vi "DP-Init Hardware.vi"(0 "State in":T2, 1 "L2":dbl format="%#_13g", 5 "freq":dbl[](array[numeric]), 7 "atten":dbl[](array[numeric]), 9 "flip":bool, 11 "error in (no error)":errorcluster, 12 "ntime":i32, 13 "nfreq":i32) -> (14 "stim":T1, 15 "error out":errorcluster)   [LabVIEW 2020]
uses:
  Typedefs/DP-Runtime State.ctl
  epl-vi-lib/Signal Synthesis VIs/4th Generation/Classes/Gate/Gate.lvclass/Gate.ctl
  e3763c63-dfad-46ca-852a-805909099497.vi
  6524839e-d3bd-4753-b68c-3c0b3b588751.vi
  epl-vi-lib/Signal Synthesis VIs/4th Generation/Common/CommonSig-Apply Ramp (2D).vi
  39a6a7b0-f891-48ff-84db-aba283587dcf.vi
  98cf35c3-bd45-4b05-b00a-4840585587a5.vi
  epl-vi-lib/Signal Synthesis VIs/4th Generation/Common/CommonSig-Apply Ramp (2D).vi/00fa021d-ebe0-42e5-9c35-5538040c7da1.vi
  epl-vi-lib/Signal Synthesis VIs/4th Generation/Classes/Gate/Write Ramp (ms).vi
  epl-vi-lib/Signal Synthesis VIs/4th Generation/Classes/Gate/Write Down (ms).vi
  epl-vi-lib/Signal Synthesis VIs/4th Generation/Classes/Gate/Write Asymmetric.vi
  epl-vi-lib/Signal Synthesis VIs/4th Generation/Classes/Gate/Write Shape.vi
  epl-vi-lib/Signal Synthesis VIs/4th Generation/Classes/Gate/Write Duration (ms).vi
  epl-vi-lib/Signal Synthesis VIs/4th Generation/Classes/Gate/Create.vi
  epl-vi-lib/Signal Synthesis VIs/4th Generation/Classes/Gate/Apply.vi
  epl-vi-lib/PXI DAQ VIs/AODO/AODO-Engine.vi
  epl-vi-lib/PXI DAQ VIs/AIDI/AIDI-Engine.vi
  <vilib>/Analysis/NI_AALBase.lvlib
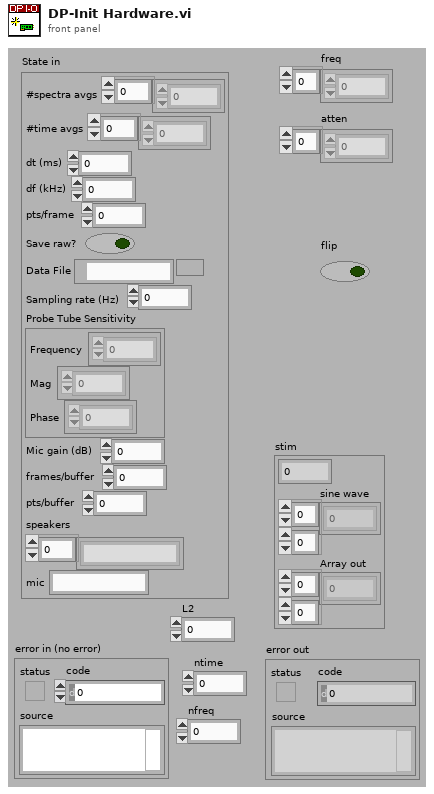
[diagram p1: front panel]
types:
  T1 = cluster{i32, "sine wave":dbl[][], "Array out":dbl[][]}
  T2 = typedef "DP-Runtime State.ctl" = cluster{"#spectra avgs":i32[], "#time avgs":i32[], "dt (ms)":dbl, "df (kHz)":dbl, "pts/frame":i32, "Save raw?":bool, "Data File":path, "Sampling rate (Hz)":dbl, "Probe Tube Sensitivity":cluster{"Frequency":dbl[], "Mag":dbl[], "Phase":dbl[]}, "Mic gain (dB)":dbl, "frames/buffer":i32, "pts/buffer":i32, "speakers":string[], "mic":string}
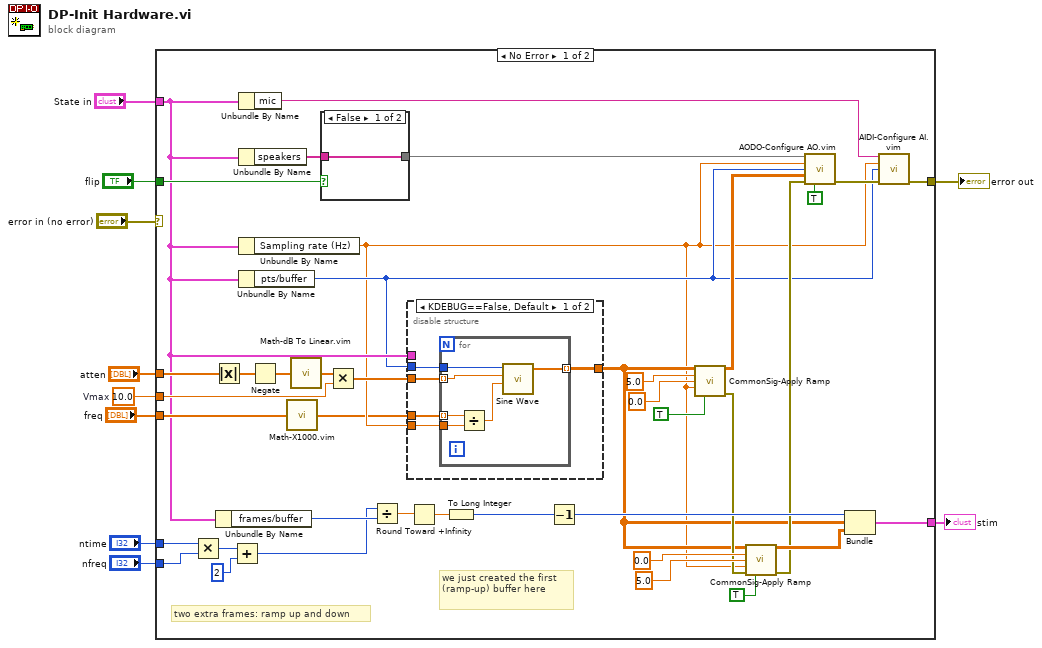
[diagram p0: block diagram]
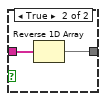
[diagram p2: hidden frame]
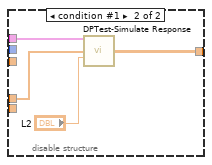
[diagram p3: hidden frame]
diagram:
  w7 = 10.0  # Vmax
  n1 = case shown="No Error" "error in (no error)" {
    selector: "error in (no error)" -> [_ w69]
    tunnel: [w50 w69] -> w10
    tunnel: "flip" -> [w48 _]
    tunnel: "State in" -> [w15 _]
    tunnel: w7 -> [w44 _]
    tunnel: "atten" -> [w43 _]
    tunnel: "freq" -> [w42 _]
    tunnel: "ntime" -> [w40 _]
    tunnel: "nfreq" -> [w39 _]
    tunnel: [w30 _] -> w1
    frame No Error {
      # "we just created the first (ramp-up) buffer here"
      # "two extra frames: ramp up and down"
      n2 = Multiply(x=w40, y=w39) -> (x*y=w38:i32)
      n3 = Absolute Value(x=w43) -> (abs(x)=w18:dbl[])
      n4 = Unbundle By Name(w15) -> ("frames/buffer"=w32:i32)
      n5 = Add(x=w38, y=2) -> (x+y=w31:i32)
      n6 = Unbundle By Name(w15) -> ("mic"=w49:string)
      n7 = Unbundle By Name(w15) -> ("speakers"=w47:string[])
      n8 = Unbundle By Name(w15) -> ("Sampling rate (Hz)"=w12:dbl)
      n9 = Unbundle By Name(w15) -> ("pts/buffer"=w13:i32)
      n10 = Negate(x=w18) -> (-x=w17:dbl[])
      n11 = call "Math-X1000.vim"("X"=w42) -> ("1000X"=w11:dbl[])
      n12 = call "Math-dB To Linear.vim"("dB"=w17) -> ("linear"=w45:dbl[])
      n13 = case shown="False" w48 {
        tunnel: w47 -> [w51 w53]
        tunnel: [w51 w52] -> w46
        frame False {
        }
        frame True {
          n14 = Reverse 1D Array(array=w53) -> (reversed array=w52:string[])
        }
      }
      n15 = Multiply(x=w45, y=w44) -> (x*y=w14:dbl[])
      n16 = Divide(x=w31, y=w32) -> (x/y=w36:dbl)
      n17 = disable-structure shown="KDEBUG==False, Default" {
        disable-tunnel: [w54 w67] -> w16
        disable-tunnel: w15 -> [_ w68]
        disable-tunnel: w11 -> [w58 w66]
        disable-tunnel: w14 -> [w57 _]
        disable-tunnel: w13 -> [w56 _]
        disable-tunnel: w12 -> [w55 _]
        frame condition #0 (active) {
          n18 = for {
            tunnel: w58 -> [w62] mode=indexing
            tunnel: w57 -> [w63] mode=indexing
            tunnel: w56 -> [w64]
            tunnel: w55 -> [w60]
            tunnel: [w59] -> w54 mode=indexing
            n19 = Divide(x=w62, y=w60) -> (x/y=w61:dbl)
            n20 = call <vilib>:"Sine Wave.vi"("samples"=w64, "amplitude"=w63, "frequency"=w61) -> ("sine wave"=w59:dbl[])  [unwired: 2 in, 2 out]
          }
        }
        frame condition #1 {
          n21 = call "DPTest-Simulate Response.vi"("state"=w68, "freqs"=w66, "L2"="L2") -> ("Stimulus out"=w67:dbl[][])  [unwired: 12 in]
        }
      }
      n22 = Round Toward +Infinity(x=w36) -> (ceil(x): smallest int >= x=w35:dbl)
      n23 = To Long Integer(number=w35) -> (32bit integer=w34:i32)
      n24 = Decrement(x=w34) -> (x-1=w33:i32)
      n25 = call-poly "CommonSig-Apply Ramp.vi"("Array in"=w16, "Ramp up (ms)"=5.0, "Ramp down (ms)"=0.0, "Fs (Hz)"=w12, "Asymmetric"=TRUE) -> ("Array out"=w41:dbl[][], "error out"=w20:errorcluster)  [unwired: 9 in]
      n26 = call-poly "CommonSig-Apply Ramp.vi"("Array in"=w16, "Ramp up (ms)"=0.0, "Ramp down (ms)"=5.0, "Fs (Hz)"=w12, "error in (no error)"=w20, "Asymmetric"=TRUE) -> ("Array out"=w24:dbl[][], "error out"=w19:errorcluster)  [unwired: 8 in]
      n27 = call "AODO-Configure AO.vim"("AO.Channels"=w46, "AO.Fs (Hz)"=w12, "AO.Npts"=w13, "AO"=w41, "error in (no error)"=w19, "Allow regen? (F)"=TRUE ("Allow regen?")) -> ("error out"=w29:errorcluster)  [unwired: 9 in]
      n28 = Bundle(w33, "sine wave"=w16, "Array out"=w24) -> (w30:T1)  [unwired: 1 in]
      n29 = call "AIDI-Configure AI.vim"("AI.Channels"=w49, "AI.Fs (Hz)"=w12, "AI.Npts"=w13, "error in (no error)"=w29) -> ("error out"=w50:errorcluster)  [unwired: 11 in]
    }
    frame Error {
    }
  }
  "error out" <- w10
  "stim" <- w1
